vi "End of Line.vi"() -> ()   [LabVIEW 2016]
panel:
  out "string out":string
  in  "string in":string
  in  "end of line (Native)":T1(ring)
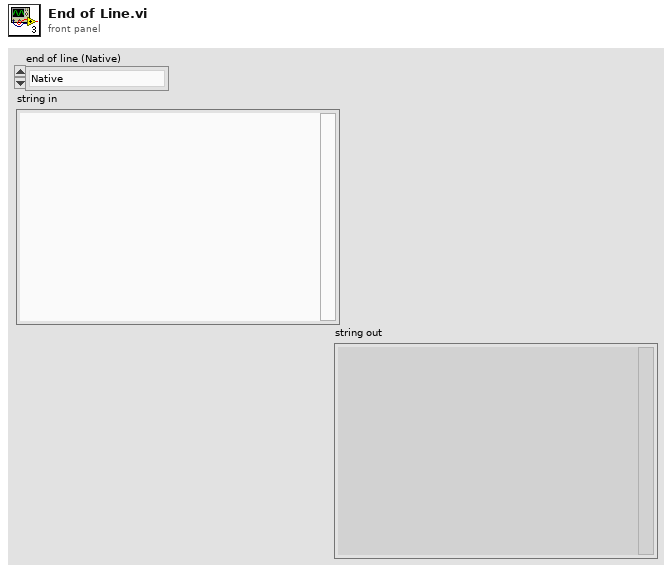
[diagram p1: front panel]
types:
  T1 = enum16{"Native", "Native Command Line", "UNIX", "Macintosh", "DOS"}
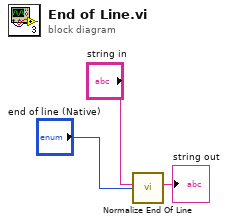
[diagram p0: block diagram]
diagram:
  n1 = call <vilib>:"Normalize End Of Line.vi"("end of line (Native)"="end of line (Native)", "string in"="string in") -> ("string out"=→"string out":string)  [unwired: 6 in]
